vi "init.vi"(8 "error in (no error)":errorcluster, 11 "EnccoderConverter in":refnum<class "EncoderConverter.lvclass">) -> (0 "error out":errorcluster, 3 "EnccoderConverter out":refnum<class "EncoderConverter.lvclass">)   [LabVIEW 2013, in "EncoderConverter.lvlib" / "EncoderConverter.lvclass"]
uses:
  <userlib>/Common/Devices/EncoderConverter/EncoderConverter/EncoderConverter.lvclass
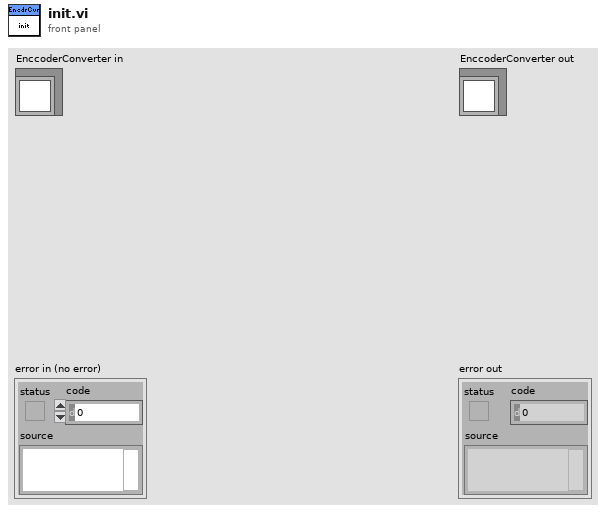
[diagram p1: front panel]
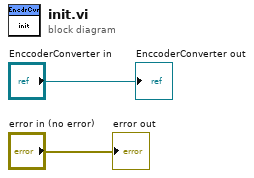
[diagram p0: block diagram]
diagram:
  "error out" <- "error in (no error)"
  "EnccoderConverter out" <- "EnccoderConverter in"
